vi "Send Message via UDP.vi"(6 "timeout ms (25000)":i32=25000, 8 "error in":errorcluster, 9 "Message":T1, 10 "Remote Port":u16, 11 "Local Port":u16) -> (0 "error out":errorcluster)   [LabVIEW 2021]
uses:
  Message.ctl
  Action.ctl
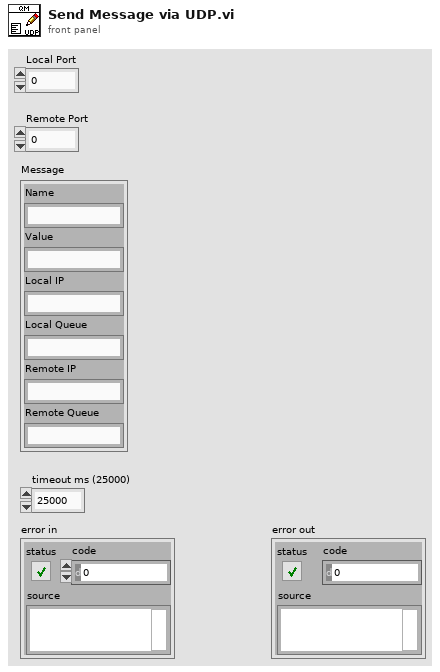
[diagram p1: front panel]
types:
  T1 = typedef "Message.ctl" = cluster{"Name":string, "Value":string, "Local IP":string, "Local Queue":string, "Remote IP":string, "Remote Queue":string}
  T2 = typedef "Action.ctl" = enum16{"Get", "Close"}
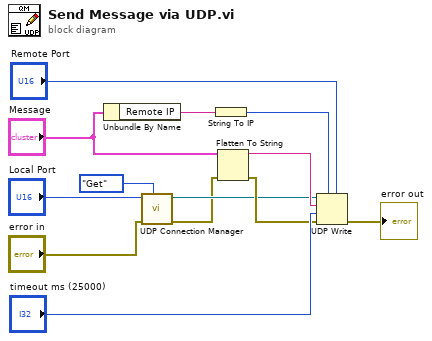
[diagram p0: block diagram]
diagram:
  n1 = Unbundle By Name("Message") -> ("Remote IP"=w7:string)
  n2 = call "UDP Connection Manager.vi"("Action"=Action."Get", "error in (no error)"="error in", "UDP Port"="Local Port") -> ("error out"=w3:errorcluster, "connection ID out"=w4:refnum<k16>)  [unwired: 7 in]
  n3 = String To IP(1:w7) -> (0:w6:u32)
  n4 = Flatten To String(anything="Message", error in (no error)=w3) -> (data string=w9:string, error out=w8:errorcluster)  [unwired: 2 in, 1 out]
  n5 = UDP Write(address=w6, port or service name="Remote Port", connection ID=w4, data in=w9, 8:w8, 9:"timeout ms (25000)") -> (error out=→"error out":errorcluster)  [unwired: 1 out]
